vi "add console output.vi"(10 "add_to_console":string) -> ()   [LabVIEW 2019, in "libSimulationControl.lvlib"]
uses:
  libSimulationControl.lvlib
panel:
  out "error out":errorcluster
  in  "error in (no error)":errorcluster
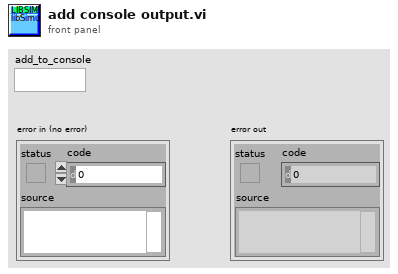
[diagram p1: front panel]
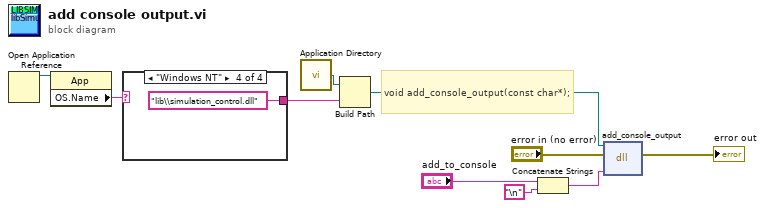
[diagram p0: block diagram]
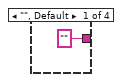
[diagram p2: hidden frame]
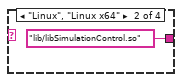
[diagram p3: hidden frame]
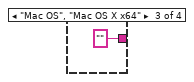
[diagram p4: hidden frame]
diagram:
  # "void add_console_output(const char*);"
  n1 = Open Application Reference() -> (3:w9:refnum<vi>)  [unwired: 4 in, 1 out]
  n2 = property class="App"(reference=w9) -> ("OS.Name"=w8:string)  [unwired: 1 in, 2 out]
  n3 = case shown="\"Windows NT\"" w8 {
    tunnel: ["" ("return type") "lib/libSimulationControl.so" ("name or relative path") "" ("return type") "lib\\simulation_control.dll" ("name or relative path")] -> w7
    frame "", Default {
    }
    frame "Linux", "Linux x64" {
    }
    frame "Mac OS", "Mac OS X x64" {
    }
    frame "Windows NT" {
    }
  }
  n4 = call <vilib>:"Application Directory.vi"() -> ("Application Directory"=w6:path)
  n5 = Build Path(base path=w6, name or relative path=w7) -> (appended path=w5:path)
  n6 = Concatenate Strings("add_to_console", "\n") -> (w1:string)
  n7 = dll-call lib="home/paul/Schreibtisch/Biogas_plant_setup/LabView/lib/libSimulationControl.so" fn="add_console_output"(path in=w5, error in="error in (no error)", "add_to_console"=w1) -> (error out=→"error out":errorcluster)  [unwired: 3 in, 1 out]
